vi "Load_Instr_Object.vi"(8 "error in (no error)":errorcluster, 9 "Instr name":string, 10 "Instr obj":refnum<class "Class Instrument (Default).lvclass">, 11 "Actor_Autotest in":refnum<class "Actor_Autotest.lvclass">) -> (0 "error out":errorcluster, 3 "Actor_Autotest out":refnum<class "Actor_Autotest.lvclass">)   [LabVIEW 2020, in "Library Core.lvlib" / "Actor_Autotest.lvlib" / "Actor_Autotest.lvclass"]
uses:
  Actor_Autotest.lvclass
  Instrument/Instrument (Default)/Class Instrument (Default).lvclass
  Actor_Autotest.lvclass/Actor_Autotest.ctl
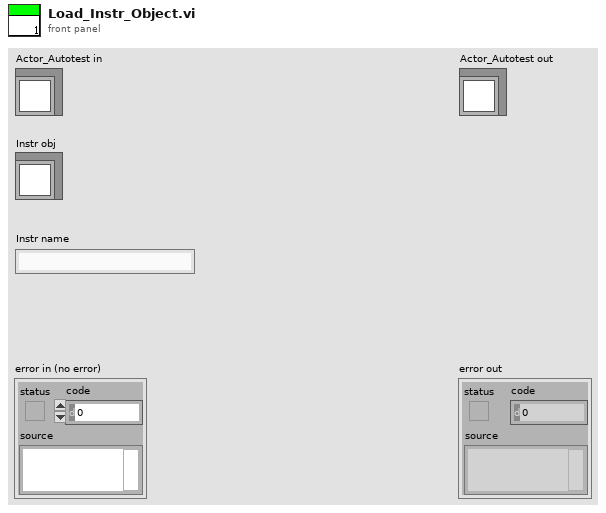
[diagram p1: front panel]
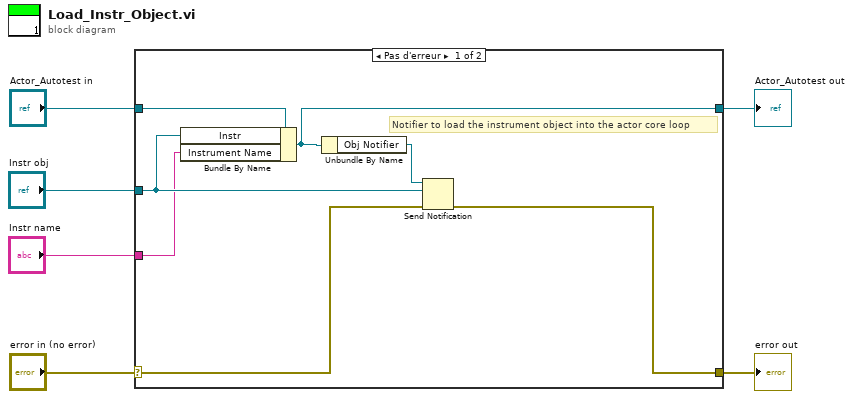
[diagram p0: block diagram]
diagram:
  n1 = case shown="Pas d'erreur" "error in (no error)" {
    selector: "error in (no error)" -> [w8 w15]
    tunnel: [w11 w15] -> w5
    tunnel: [w9 w14] -> w3
    tunnel: "Actor_Autotest in" -> [w13 w14]
    tunnel: "Instr obj" -> [w12 _]
    tunnel: "Instr name" -> [w10 _]
    frame No Error {
      # "Notifier to load the instrument object into the actor core loop"
      n2 = Bundle By Name(cluster=w13, "Instr"=w12, "Instrument Name"=w10) -> (w9:refnum<class "Actor_Autotest.lvclass">)
      n3 = Unbundle By Name(w9) -> ("Obj Notifier"=w7:refnum<notifier>)
      n4 = Send Notification(notification=w12, notifier=w7, error in (no error)=w8) -> (error out=w11:errorcluster)  [unwired: 1 out]
    }
    frame Error {
    }
  }
  "error out" <- w5
  "Actor_Autotest out" <- w3
